vi "Client.vi"() -> ()   [LabVIEW 2021]
panel:
  in  "stop":bool
  in  "C6":bool
  in  "C5":bool
  in  "C4":bool
  in  "C3":bool
  in  "C2":bool
  in  "C1":bool
  in  "B6":bool
  in  "B5":bool
  in  "B4":bool
  in  "B3":bool
  in  "B2":bool
  in  "B1":bool
  in  "A6":bool
  in  "A5":bool
  in  "A4":bool
  in  "A3":bool
  in  "A2":bool
  in  "A1":bool
  # "1"
  # "2"
  # "3"
  # "4"
  # "5"
  # "6"
  # "Alarm Switches"
  # "Bypass Switches"
  # "Tamper Switches"
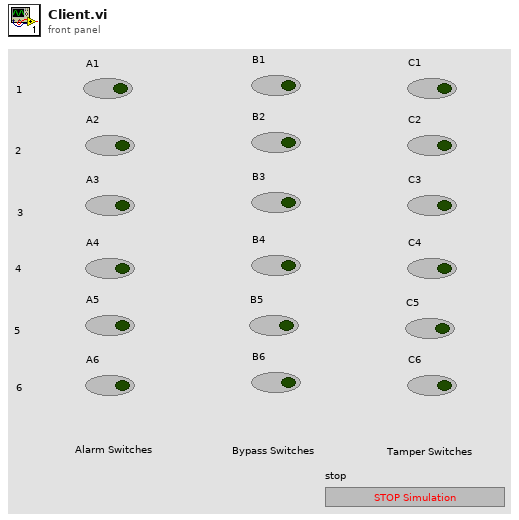
[diagram p1: front panel]
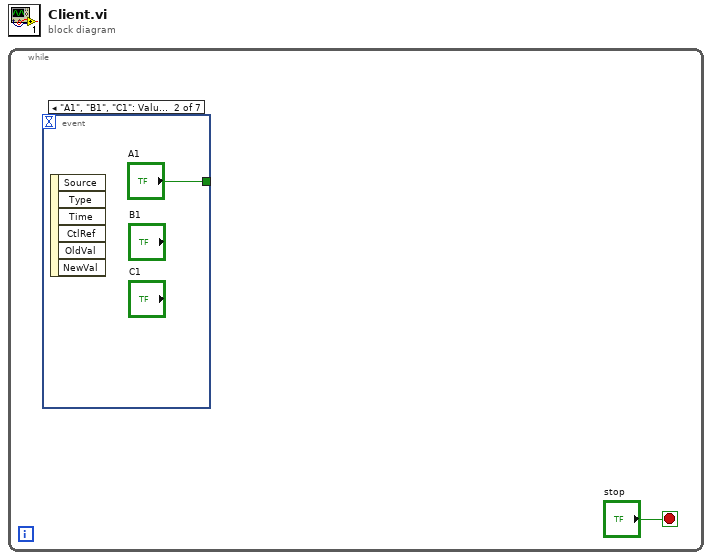
[diagram p0: block diagram]
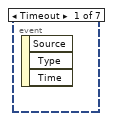
[diagram p2: hidden frame]
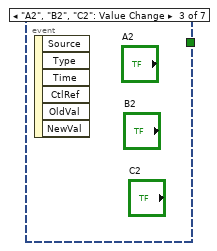
[diagram p3: hidden frame]
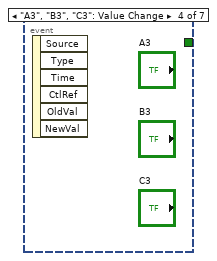
[diagram p4: hidden frame]
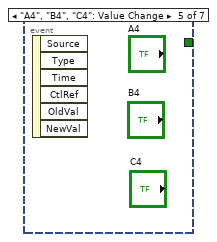
[diagram p5: hidden frame]
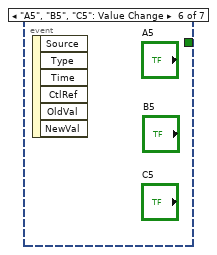
[diagram p6: hidden frame]
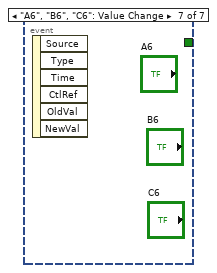
[diagram p7: hidden frame]
diagram:
  n1 = while {
    stop <- "stop" stop-if-true
    n2 = event shown="[1] \"A1\", \"B1\", \"C1\": Value Change" {
      selector: _ -> [_ _ _ _ _ _ _]
      dyn-events: _ -> [_ _ _ _ _ _ _]
      timeout: _ -> [_ _ _ _ _ _ _]
      tunnel: [_ "A1" _ _ _ _ _] -> _
      event Timeout {
        n3 = event-data() -> ()  [unwired: 1 in, 3 out]
      }
      event "A1", "B1", "C1": Value Change {
        n4 = event-data() -> ()  [unwired: 1 in, 6 out]
      }
      event "A2", "B2", "C2": Value Change {
        n5 = event-data() -> ()  [unwired: 1 in, 6 out]
      }
      event "A3", "B3", "C3": Value Change {
        n6 = event-data() -> ()  [unwired: 1 in, 6 out]
      }
      event "A4", "B4", "C4": Value Change {
        n7 = event-data() -> ()  [unwired: 1 in, 6 out]
      }
      event "A5", "B5", "C5": Value Change {
        n8 = event-data() -> ()  [unwired: 1 in, 6 out]
      }
      event "A6", "B6", "C6": Value Change {
        n9 = event-data() -> ()  [unwired: 1 in, 6 out]
      }
    }
  }
